vi "RIOduino_Begin.vi"   [LabVIEW 2015]
uses:
  <vilib>/Rock Robotics/SystemInterfaces/i2clib/i2c_bus.ctl
types:
  T1 = typedef "i2c_bus.ctl" = enum16{"I2C On-Board", "I2C MXP", "Invalid"}
  T2 = typedef "WPI_I2CDevRef.ctl" = cluster{"DevStatus":errorcluster, "Device Address":u8, "Handle":i32, "I2C Bus":T1}
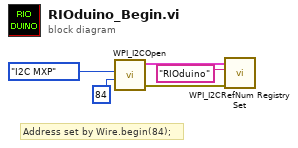
[diagram p0: block diagram]
diagram:
  # "Address set by Wire.begin(84);"
  n1 = call <vilib>:"WPI_I2COpen.vi"("Device Address"=u8 84, "I2C Bus"=i2c_bus."I2C MXP") -> ("error out"=w3:errorcluster, "I2CDevRef"=w2:T2)  [unwired: 8 in]
  n2 = call <vilib>:"WPI_I2CRefNum Registry Set.vi"("error in (no error)"=w3, "refnum name"="RIOduino", "I2CDevRef"=w2) -> ()  [unwired: 7 in, 2 out]
